vi "Patch data preview-Set pos scrollbar limits.vi"(8 "error in (no error)":errorcluster, 10 "Last cycle's number":i32, 11 "Scrollbar":refnum<vi>) -> (0 "error out":errorcluster, 3 "Scrollbar":refnum<vi>)   [LabVIEW 2017]
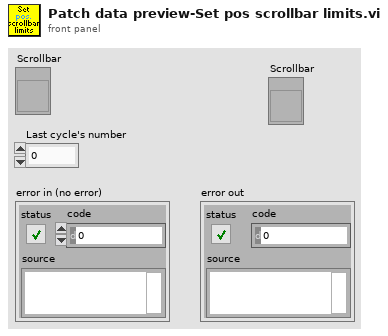
[diagram p1: front panel]
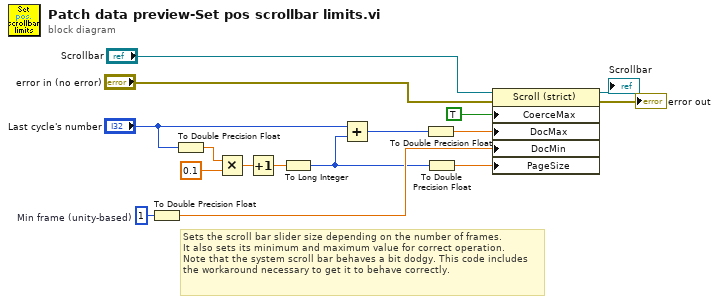
[diagram p0: block diagram]
diagram:
  w15 = u32 1  # Min frame (unity-based)
  # "Sets the scroll bar slider size depending on the number of frames.\nIt also sets its minimum and maximum value for correct operation.\nNote that the system scroll bar behaves a bit dodgy. This code includes the workaround necessary to get it to behave correctly."
  n1 = To Double Precision Float(number=w15) -> (double precision float=w9:dbl)
  n2 = To Double Precision Float(number="Last cycle's number") -> (double precision float=w16:dbl)
  n3 = Multiply(x=w16, y=0.1) -> (x*y=w11:dbl)
  n4 = Increment(x=w11) -> (x+1=w13:dbl)
  n5 = To Long Integer(number=w13) -> (32bit integer=w5:i32)
  n6 = Add(x="Last cycle's number", y=w5) -> (x+y=w1:i32)
  n7 = To Double Precision Float(number=w1) -> (double precision float=w3:dbl)
  n8 = To Double Precision Float(number=w5) -> (double precision float=w2:dbl)
  n9 = property on="Property Node" class="Scroll (strict)"(reference="Scrollbar", error in="error in (no error)", "CoerceMax"=TRUE ("Coerce Maximum Value"), "DocMax"=w3, "DocMin"=w9, "PageSize"=w2) -> (reference out=→"Scrollbar":refnum<vi>, error out=→"error out":errorcluster)
